vi "FramePack.vi"(4 "ADataArray":u8[](array[numeric]), 6 "ADLC":u8, 7 "AID":u32, 9 "AIsRemote":enum16{"数据帧", "远程帧"}(ring), 10 "AIsExt":enum16{"标准帧", "扩展帧"}(ring)) -> (2 "CANframe":T1 {"ADLC" max=64; "AID" max=536870911})   [LabVIEW 2016]
uses:
  Ctrl/CAN_FrameInfo.ctl
panel:
  in  "发送数据帧信息":T1={"AID"=1234, "AIsExt"=enum."STD", "AIsRemote"=enum."Data", "ADLC"=5, "ADataArray"=[0, 0, 10, 96, 8, 8]} {"ADLC" max=64; "AID" max=536870911}
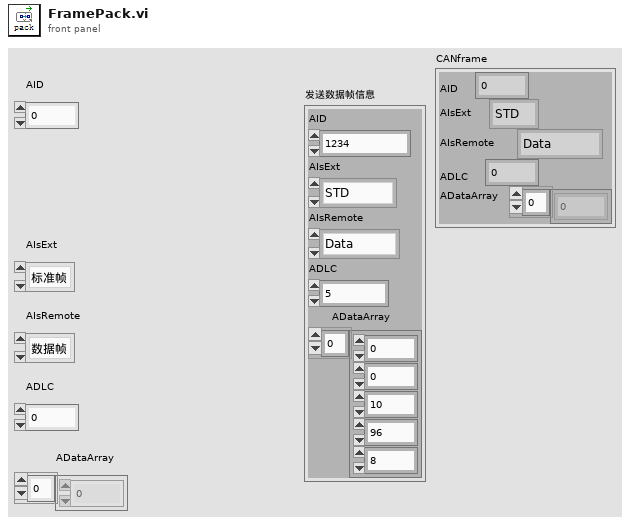
[diagram p1: front panel]
types:
  T1 = typedef "CAN_FrameInfo.ctl" = cluster{"AID":u32, "AIsExt":enum16{"STD", "EXT"}, "AIsRemote":enum16{"Data", "Remote"}, "ADLC":u8, "ADataArray":u8[]}
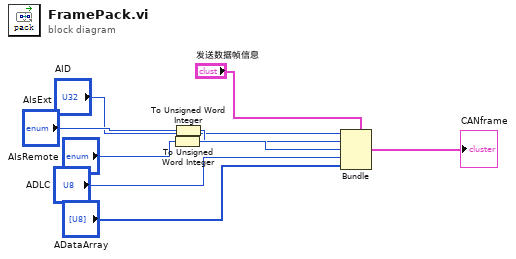
[diagram p0: block diagram]
diagram:
  n1 = To Unsigned Word Integer(number="AIsRemote") -> (unsigned 16bit integer=w6:u16)
  n2 = To Unsigned Word Integer(number="AIsExt") -> (unsigned 16bit integer=w5:u16)
  n3 = Bundle(cluster="发送数据帧信息", "AID"="AID", "AIsExt"=w5, "AIsRemote"=w6, "ADLC"="ADLC", "ADataArray"="ADataArray") -> (→"CANframe":T1)
